vi "Send MSG.vi"(0 "CAN Channel Handle":u32, 1 "Arbitration ID":u32=100, 2 "Packet":u8[](array[numeric])=[103, 82, 84, 0, 0, 0, 0, 0]) -> ()   [LabVIEW 2011]
panel:
  out "Send OK":bool
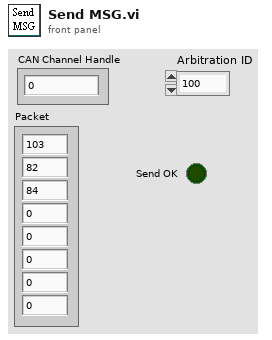
[diagram p1: front panel]
types:
  T1 = cluster{"Timestamp":u32, "Arbitration ID":u32, "DLC":u8, "Type":u8, "extended frame":bool, "remote request":bool, "self reception":bool, "Data":cluster{"[0]":u8, "[1]":u8, "[2]":u8, "[3]":u8, "[4]":u8, "[5]":u8, "[6]":u8, "[7]":u8}}
  T2 = cluster{"Packet[0]":u8, "Packet[1]":u8, "Packet[2]":u8, "Packet[3]":u8, "Packet[4]":u8, "Packet[5]":u8, "Packet[6]":u8, "Packet[7]":u8}
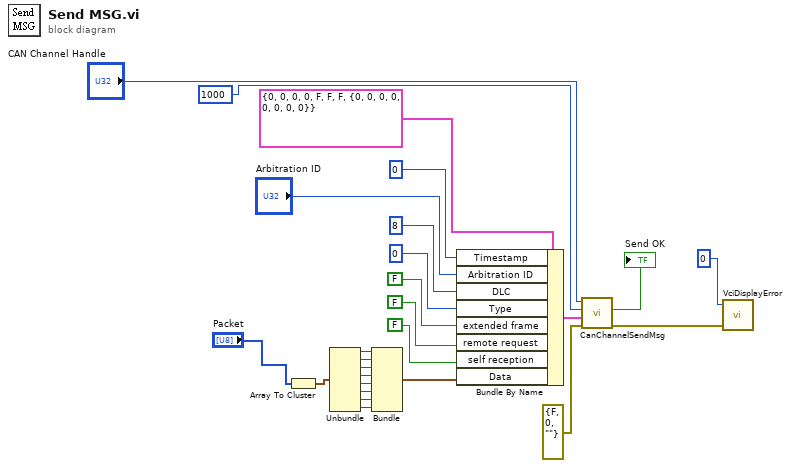
[diagram p0: block diagram]
diagram:
  n1 = Array To Cluster(array="Packet") -> (cluster=w11:T2)
  n2 = Unbundle(w11) -> ("Packet[0]"=w10:u8, "Packet[1]"=w9:u8, "Packet[2]"=w8:u8, "Packet[3]"=w7:u8, "Packet[4]"=w6:u8, "Packet[5]"=w5:u8, "Packet[6]"=w4:u8, "Packet[7]"=w3:u8)
  n3 = Bundle("Packet[0]"=w10, "Packet[1]"=w9, "Packet[2]"=w8, "Packet[3]"=w7, "Packet[4]"=w6, "Packet[5]"=w5, "Packet[6]"=w4, "Packet[7]"=w3) -> (w13:T2)  [unwired: 1 in]
  n4 = Bundle By Name(cluster=T1 {"Timestamp"=0, "Arbitration ID"=0, "DLC"=0, "Type"=0, "extended frame"=FALSE, "remote request"=FALSE, "self reception"=FALSE, "Data"={"[0]"=0, "[1]"=0, "[2]"=0, "[3]"=0, "[4]"=0, "[5]"=0, "[6]"=0, "[7]"=0}} ("CAN message"), "Timestamp"=u32 0, "Arbitration ID"="Arbitration ID", "DLC"=u8 8, "Type"=u8 0, "extended frame"=FALSE, "remote request"=FALSE, "self reception"=FALSE, "Data"=w13) -> (w15:T1)
  n5 = call "CanChannelSendMsg.vi"("error in"=errorcluster {"status"=FALSE, "code"=0, "source"=""}, "CAN message"=w15, "Milliseconds"=u32 1000, "CAN Channel Handle in"="CAN Channel Handle") -> ("error out"=w18:errorcluster, "Send OK"=→"Send OK":bool)  [unwired: 1 in, 1 out]
  n6 = call "VciDisplayError.vi"("error in"=w18, "HWND Parent"=u32 0) -> ()  [unwired: 4 in]
